vi "Loop.vi"   [LabVIEW 2016, in "Test.lvrbt"]
uses:
  Test.lvrbt
  <vilib>/NXT/Block Support/NXT_OutputPort.ctl
  <vilib>/NXT/LegoClasses/BrickReference/BrickReference.lvclass
  <vilib>/NXT/Subs/LVHSConnector.ctl
  <vilib>/NXT/NXTIO Xnodes/NXTIONodeSubVIs/NXTMoveMotors.vi
  <vilib>/NXT/NXTIO Xnodes/NXTIOXNode/NXTIO.xnode
  <vilib>/NXT/NXTIO Xnodes/AddressXNode/NXTIOAddress.xnode
  <vilib>/NXT/Dual Mode Library/Waits/Wait_Num.vi
  <vilib>/NXT/NXTIO Xnodes/NXTIONodeSubVIs/NXTStopMotors.vi
  <vilib>/NXT/Dual Mode Library/Sound/Tone.vi
  <vilib>/NXT/Dual Mode Library/Waits/Wait_Touch.vi
  <vilib>/NXT/Block Support/NXT_InputPort.ctl
types:
  T1 = typedef "NXT_OutputPort.ctl" = u8
  T2 = typedef "LVHSConnector.ctl" = refnum<class "BrickReference.lvclass">
  T3 = typedef "NXT_InputPort.ctl" = u32
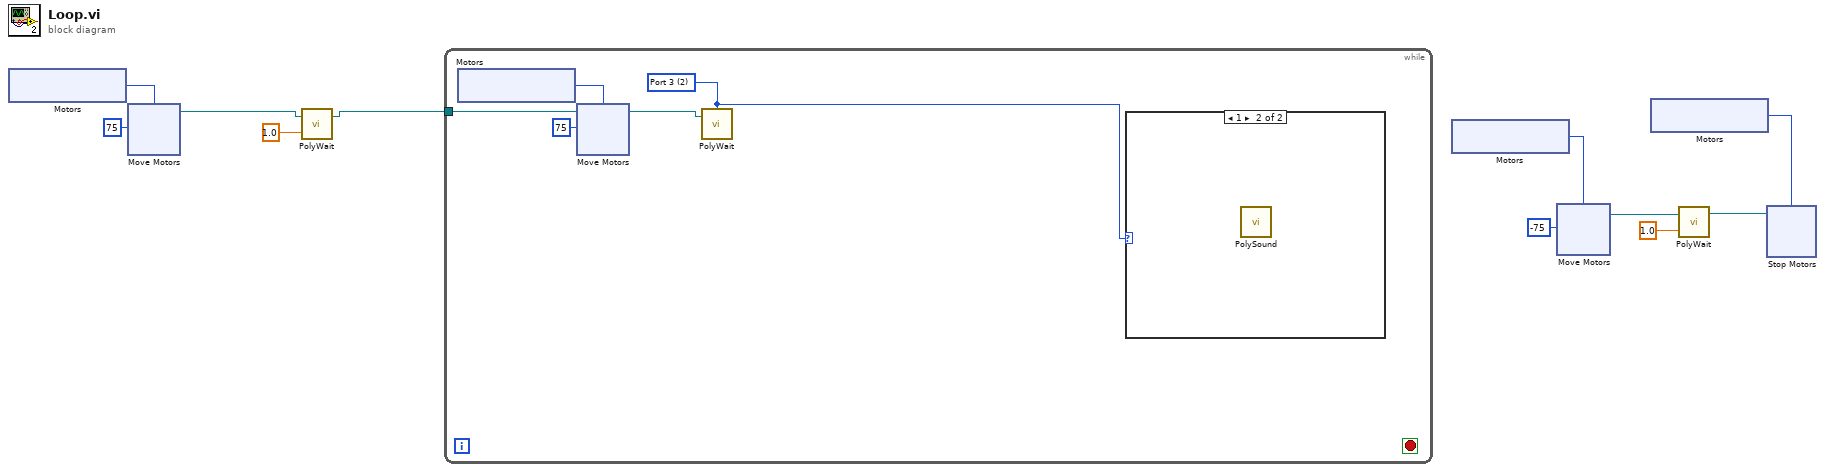
[diagram p0: block diagram]
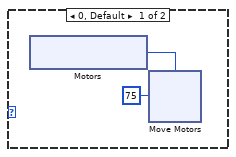
[diagram p2: hidden frame]
diagram:
  n1 = xnode "Motors"() -> ("Motor"=w11:T1)
  n2 = xnode "Move Motors"("Power/Speed 1"=i8 75, "Motors"=w11) -> ("NXT/EV3"=w9:T2)  [unwired: 1 in]
  n3 = call-poly <vilib>:"PolyWait.vi"("Time (1 sec)"=sgl 1.0, "NXT/EV3"=w9) -> ("NXT/EV3"=w1:T2)  [unwired: 2 in]
  n4 = while {
    tunnel: w1 -> [w14]
    stop <- _ stop-if-true
    w12 = T3 2 items=["Port 1", "Port 2", "Port 3", "Port 4"] ("Port (Port 1)")
    n5 = xnode "Motors"() -> ("Motor"=w16:T1)
    n6 = xnode "Move Motors"("Power/Speed 1"=i8 75, "Motors"=w16, "NXT/EV3"=w14) -> ("NXT/EV3"=w13:T2)
    n7 = call-poly <vilib>:"PolyWait.vi"("NXT/EV3"=w13, "Port (Port 1)"=w12) -> ()  [unwired: 2 in, 1 out]
    n8 = case shown="1" w12 {
      frame 0, Default {
        n9 = xnode "Motors"() -> ("Motor"=w18:T1)
        n10 = xnode "Move Motors"("Power/Speed 1"=i8 75, "Motors"=w18) -> ()  [unwired: 1 in, 1 out]
      }
      frame 1 {
        n11 = call-poly <vilib>:"PolySound.vi"() -> ()  [unwired: 4 in, 1 out]
      }
    }
  }
  n12 = xnode "Motors"() -> ("Motor"=w7:T1)
  n13 = xnode "Move Motors"("Power/Speed 1"=i8 -75, "Motors"=w7) -> ("NXT/EV3"=w4:T2)  [unwired: 1 in]
  n14 = xnode "Motors"() -> ("Motor"=w2:T1)
  n15 = call-poly <vilib>:"PolyWait.vi"("Time (1 sec)"=sgl 1.0, "NXT/EV3"=w4) -> ("NXT/EV3"=w3:T2)  [unwired: 2 in]
  n16 = xnode "Stop Motors"("Motors"=w2, "NXT/EV3"=w3) -> ()  [unwired: 1 out]
